vi "Update Active Attribute Value.vi"(8 "error in (no error)":errorcluster, 10 "Data":variant, 11 "Edit Sequence Dialog in":refnum<class "Subroutine Dialog.lvclass">) -> (0 "error out":errorcluster, 3 "Edit Sequence Dialog out":refnum<class "Subroutine Dialog.lvclass">)   [LabVIEW 2017, in "Subroutine Dialog.lvclass"]
uses:
  <vilib>/gpm_packages/@cs/Test-executive-builder/Source/Test Executive Builder Dialogs/Edit Subroutine Dialog/Subroutine Dialog.lvclass
  <vilib>/gpm_packages/@cs/Test-executive-builder/Source/Test Executive Builder Dialogs/Edit Subroutine Dialog/Subroutine Dialog.lvclass/Subroutine Dialog.ctl
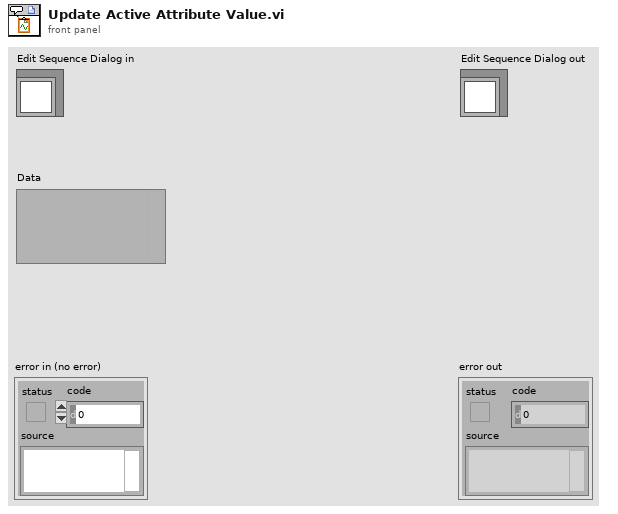
[diagram p1: front panel]
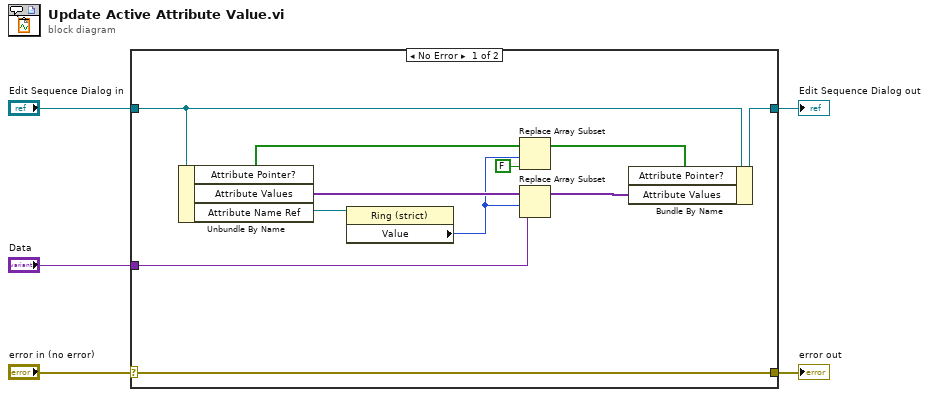
[diagram p0: block diagram]
diagram:
  n1 = case shown="No Error" "error in (no error)" {
    selector: "error in (no error)" -> [w16 w18]
    tunnel: [w16 w18] -> w4
    tunnel: [w11 w17] -> w2
    tunnel: "Edit Sequence Dialog in" -> [w12 w17]
    tunnel: "Data" -> [w13 _]
    frame No Error {
      n2 = Unbundle By Name(w12) -> ("Attribute Pointer?"=w9:bool[], "Attribute Values"=w14:variant[], "Attribute Name Ref"=w15:refnum<vi>)
      n3 = property class="Ring (strict)"(reference=w15) -> ("Value"=w7:u16)  [unwired: 1 in, 2 out]
      n4 = Replace Array Subset(array=w9, new element=FALSE ("new element/subarray"), index=w7) -> (w8:bool[])
      n5 = Replace Array Subset(array=w14, new element=w13, index=w7) -> (w10:variant[])
      n6 = Bundle By Name(cluster=w12, "Attribute Pointer?"=w8, "Attribute Values"=w10) -> (w11:refnum<class "Subroutine Dialog.lvclass">)
    }
    frame Error {
    }
  }
  "error out" <- w4
  "Edit Sequence Dialog out" <- w2
